vi "SQ Lite Prepare Cluster_WPX.vi"() -> ()   [LabVIEW 2017]
uses:
  <vilib>/Utility/Data Type/NI_Data Type.lvlib
  SQ Lite Cluster Action.ctl
  Beltwatch/BeltWatch 4-2-2-5/Database/Beltwatch SQLite.lvlib
  Beltwatch/BeltWatch 4-2-2-5/BeltWatch Event type.ctl
  Beltwatch/BeltWatch 4-2-2-5/BeltWatch Alarm Priority.ctl
  Beltwatch/BeltWatch 4-2-2-5/BeltWatch Reading.ctl
  Beltwatch/BeltWatch 4-2-2-5/Overlay mode.ctl
  Beltwatch/BeltWatch 4-2-2-5/BeltWatch 2D overlay.ctl
  Beltwatch/BeltWatch 4-2-2-5/Events class.ctl
  Beltwatch/BeltWatch 4-2-2-5/BeltWatch Event.ctl
  <vilib>/Utility/Data Type/Type Definitions/Data Type.ctl
panel:
  out "Array 4":u32[](array[numeric])
  out "Array 3":string[][](array[string])
  in  "Readings":T1[](array[typedef])=[{"Reading #"=0, "Readings"=[3.9289019107818604], "Reading Name"="Splice distortion", "Type"=enum."Defect", "Alarm priority"=enum."No Alarm", "Display precision"=0}, {"Reading #"=1, "Readings"=[1328.95654296875], "Reading Name"="Splice length", "Type"=enum."Defect", "Alarm priority"=enum."No Alarm", "Display precision"=0}, {"Reading #"=2, "Readings"=[0.0], "Reading Name"="Splice necking", "Type"=enum."Defect", "Alarm priority"=enum."No Alarm", "Display precision"=0}, {"Reading #"=3, "Readings"=[0.0], "Reading Name"="Splice Max Amplitude ", "Type"=enum."Defect", "Alarm priority"=enum."No Alarm", "Display precision"=0}, {"Reading #"=4, "Readings"=[0.0], "Reading Name"="Width at Splice", "Type"=enum."Defect", "Alarm priority"=enum."No Alarm", "Display precision"=0}, {"Reading #"=5, "Readings"=[0.0], "Reading Name"="Tracking at splice", "Type"=enum."Defect", "Alarm priority"=enum."No Alarm", "Display precision"=0}, {"Reading #"=0, "Readings"=[2.0], "Reading Name"="No. Breaks", "Type"=enum."Defect", "Alarm priority"=enum."No Alarm", "Display precision"=0}, {"Reading #"=1, "Readings"=[7.372896194458008], "Reading Name"="Max  Amplitude (V)", "Type"=enum."Defect", "Alarm priority"=enum."No Alarm", "Display precision"=0}, {"Reading #"=2, "Readings"=[10.810811042785645], "Reading Name"="% Belt Width", "Type"=enum."Defect", "Alarm priority"=enum."No Alarm", "Display precision"=0}, {"Reading #"=3, "Readings"=[0.0], "Reading Name"="% Center Width (%)", "Type"=enum."Defect", "Alarm priority"=enum."No Alarm", "Display precision"=0}, {"Reading #"=4, "Readings"=[0.0], "Reading Name"=" % Max Edge Width", "Type"=enum."Defect", "Alarm priority"=enum."No Alarm", "Display precision"=0}]
  out "element action":T4[](array[typedef])
  in  "Cluster":cluster{"Include":bool, "Name":string}={"Include"=TRUE, "Name"=""}
  in  "String":string
  out "Cluster Elements":variant[](array[variant])
  out "Array 2":string[](array[string])
  out "Array":T5[](array[typedef])
  in  "Event Out":T6
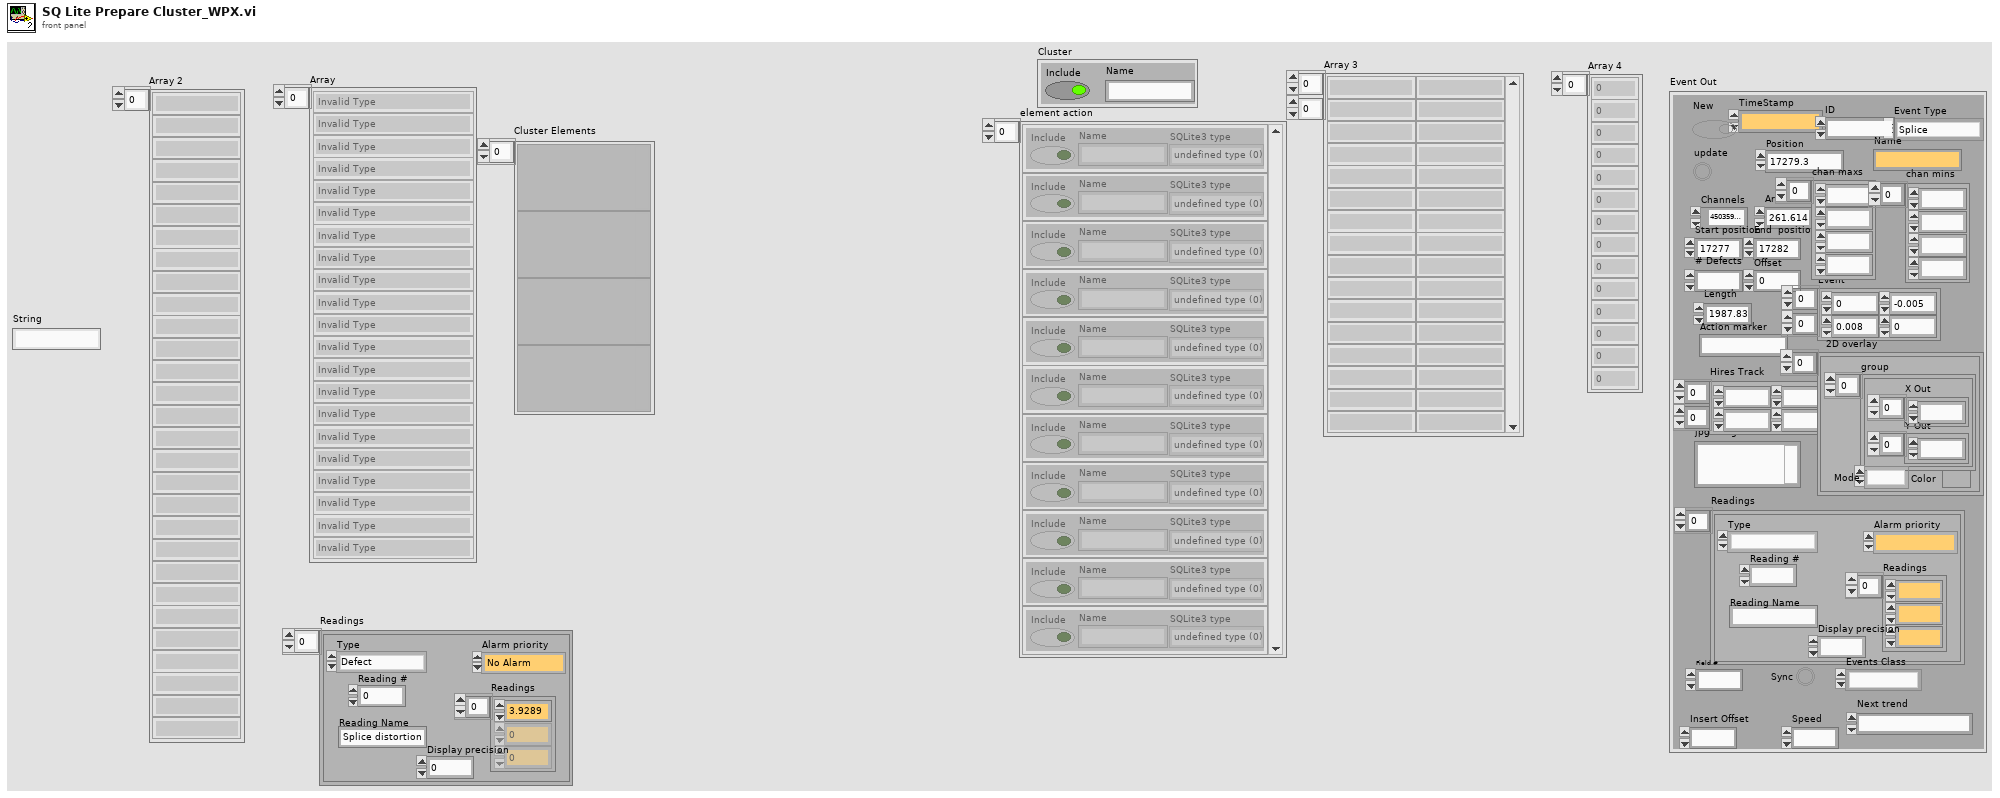
[diagram p1: front panel]
types:
  T1 = typedef "BeltWatch Reading.ctl" = cluster{"Reading #":i32, "Readings":dbl[], "Reading Name":string, "Type":T2, "Alarm priority":T3, "Display precision":i32}
  T2 = typedef "BeltWatch Event type.ctl" = enum16{"Defect", "Splice", "Break", "Rip", "Track", "Segment", "Belt", "New Splice", "Missing Splice", "None", "Free"}
  T3 = typedef "BeltWatch Alarm Priority.ctl" = enum16{"No Alarm", "High", "Medium", "Low"}
  T4 = typedef "Beltwatch SQLite.lvlib/SQ Lite Cluster Action.ctl" = cluster{"Include":bool, "Name":string, "SQLite3 type":enum32{"undefined type (0)", "SQLITE_INTEGER", "SQLITE_FLOAT", "SQLITE3_TEXT", "SQLITE_BLOB", "SQLITE_NULL", "undefined type"}}
  T5 = typedef "NI_Data Type.lvlib/Data Type.ctl" = enum8{"Invalid Type", "Void", "I8", "I16", "I32", "I64", "U8", "U16", "U32", "U64", "Single Float", "Double Float", "Extended Float", "Single Complex", "Double Complex", "Extended Complex", "Enum U8", "Enum U16", "Enum U32", "Enum U64", "Single Float With Unit", "Double Float With Unit", "Extended Float With Unit", "Single Complex with Unit", "Double Complex with Unit", "Extended Complex with Unit", "Boolean", "String", "Path", "Picture", "Tag", "Array", "Cluster", "Variant", "LV Variant", "Waveform", "Timestamp", "Digital Waveform", "Digital Data", "ExpressData", "Refnum", "External Data", "VI", "Poly VI", "LabVIEW Class Instance", "Fixed Point"}
  T6 = typedef "BeltWatch Event.ctl" = cluster{"Position":dbl, "Event Type":T2, "Area":dbl, "Channels":u64, "Start position":dbl, "End  position":dbl, "Name":string, "Offset":dbl, "Length":dbl, "Action marker":string, "Event":dbl[][], "# Defects":i32, "jpg Image":string, "chan maxs":dbl[], "chan mins":dbl[], "TimeStamp":dbl, "Readings":T1[], "ID":u32, "New":bool, "Hires Track":dbl[][], "2D overlay":T7, "update":bool, "Field #":i32, "Events Class":T9, "Sync":bool, "Insert Offset":dbl, "Next trend":dbl, "Speed":dbl}
  T7 = typedef "BeltWatch 2D overlay.ctl" = cluster{"group":cluster{"X Out":sgl[], "Y Out":sgl[]}[], "Color ":u32, "Mode":T8}[]
  T8 = typedef "Overlay mode.ctl" = enum16{"Line", "point", "Box", "Oval", "Numbannotation"}
  T9 = typedef "Events class.ctl" = enum16{"Reference", "Inspection", "New", "Tramp", "Align", "Ready"}
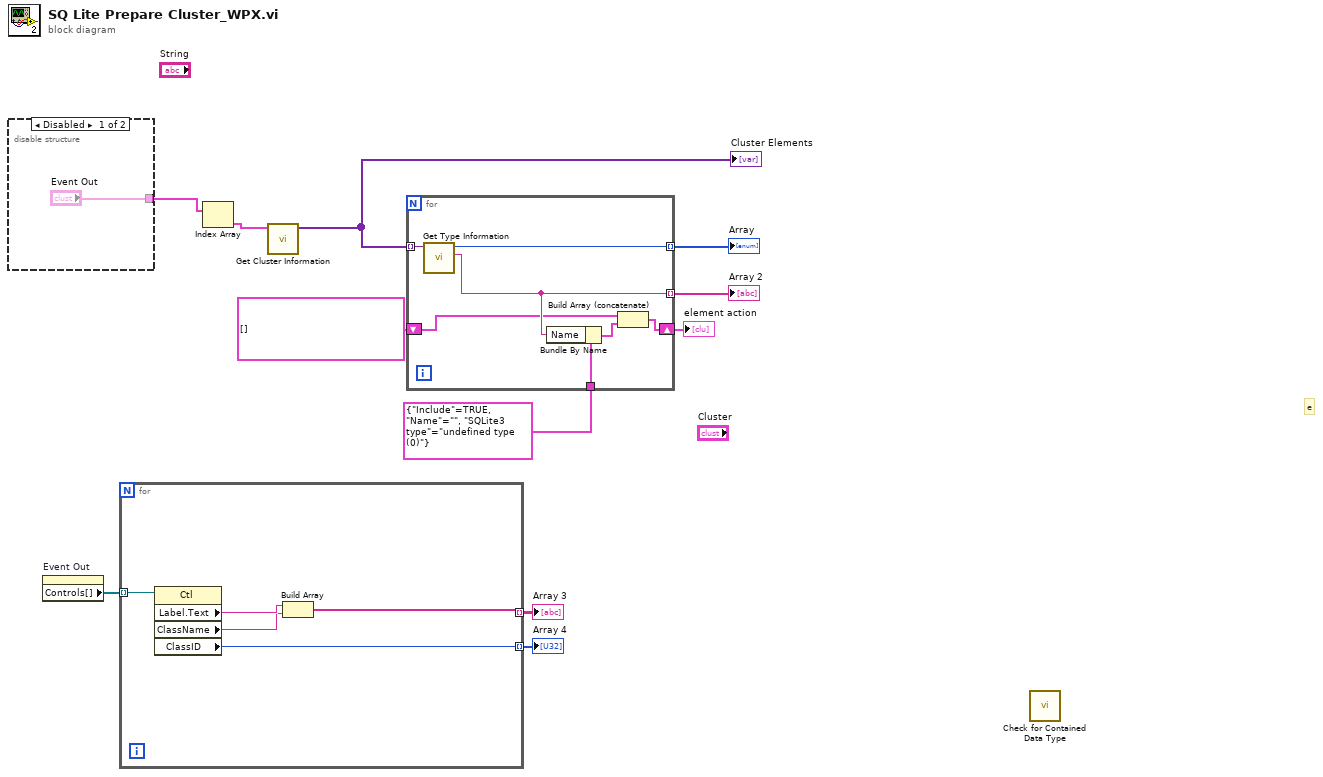
[diagram p0: block diagram]
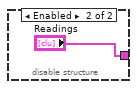
[diagram p2: hidden frame]
diagram:
  # "e"
  n1 = disable-structure shown="Disabled" {
    disable-tunnel: ["Event Out" "Readings"] -> w5
    frame Disabled {
    }
    frame Enabled {
    }
  }
  n2 = property on="Event Out" class="Clust (strict)"() -> ("Controls[]"=w3:refnum<vi>[])  [unwired: 2 in, 2 out]
  n3 = for {
    tunnel: w3 -> [w18] mode=indexing
    tunnel: [w15] -> w2 mode=indexing
    tunnel: [w14] -> w1 mode=indexing
    n4 = property class="Ctl"(reference=w18) -> ("Label.Text"=w17:string, "ClassName"=w16:string, "ClassID"=w14:u32)  [unwired: 1 in, 2 out]
    n5 = Build Array(w17, w16) -> (w15:string[])
  }
  "Array 3" <- w2
  "Array 4" <- w1
  n6 = Index Array(array=w5) -> (element=w4:T1)  [unwired: 1 in]
  n7 = call <vilib>:"Get Cluster Information.vi"("Variant"=w4) -> ("Cluster Elements"=w11:variant[])  [unwired: 9 in, 1 out]
  "Cluster Elements" <- w11
  n8 = for {
    tunnel: w11 -> [w25] mode=indexing
    tunnel: [w24] -> w10 mode=indexing
    shift-right: [w20] -> w6
    shift-left: T4[] [] -> [w19]
    tunnel: T4 {"Include"=TRUE, "Name"="", "SQLite3 type"=enum."undefined type (0)"} ("Cluster") -> [w23]
    tunnel: [w21] -> w8 mode=indexing
    n9 = call <vilib>:"Get Type Information.vi"("Variant"=w25) -> ("Name"=w21:string, "Type"=w24:T5)  [unwired: 6 in, 3 out]
    n10 = Bundle By Name(cluster=w23, "Name"=w21) -> (w22:T4)
    n11 = Build Array (concatenate)(w19, w22) -> (w20:T4[])
  }
  "Array" <- w10
  "Array 2" <- w8
  "element action" <- w6
  n12 = call <vilib>:"Check for Contained Data Type.vi"() -> ()  [unwired: 10 in, 2 out]
